vi "SweepGen.vi"(0 "#pts2":u32=21, 2 "#pts1":u32=21, 3 "Stop2":dbl=10.0 format="%.3p", 4 "Start2":dbl format="%.3p", 5 "Stop1":dbl=10.0 format="%.3p", 6 "Start1":dbl format="%.3p") -> (1 "Sweep":cluster{dbl[], dbl[]}(graph))   [LabVIEW 2022 SP3]
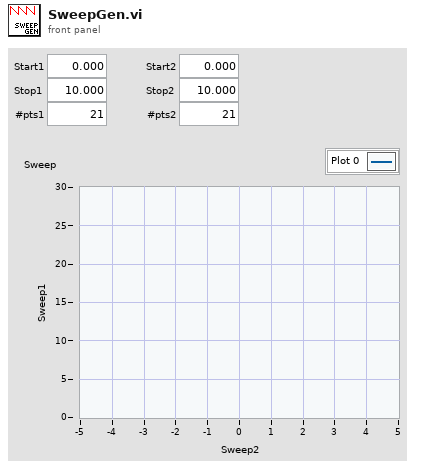
[diagram p1: front panel]
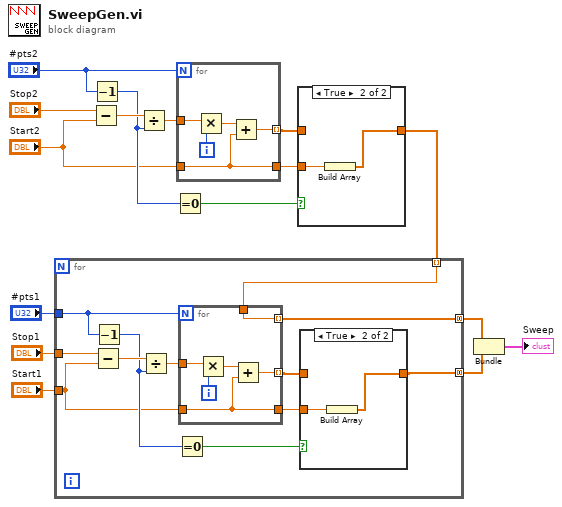
[diagram p0: block diagram]
diagram:
  n1 = Subtract(x="Stop2", y="Start2") -> (x-y=w16:dbl)
  n2 = Decrement(x="#pts2") -> (x-1=w14:u32)
  n3 = Divide(x=w16, y=w14) -> (x/y=w15:dbl)
  n4 = Equal To 0?(x=w14) -> (x = 0?=w10:bool)
  n5 = for {
    N: "#pts2" -> [_]
    tunnel: w15 -> [w21]
    tunnel: "Start2" -> [w17]
    tunnel: [w18] -> w9 mode=indexing
    tunnel: [w17] -> w8
    i -> [w20]
    n6 = Multiply(x=w21, y=w20) -> (x*y=w19:dbl)
    n7 = Add(x=w19, y=w17) -> (x+y=w18:dbl)
  }
  n8 = case shown="True" w10 {
    tunnel: [w22 w23] -> w4
    tunnel: w9 -> [w22 _]
    tunnel: w8 -> [_ w24]
    frame False {
    }
    frame True {
      n9 = Build Array(w24) -> (w23:dbl[])
    }
  }
  n10 = for {
    tunnel: "#pts1" -> [w33]
    tunnel: "Stop1" -> [w32]
    tunnel: "Start1" -> [w31]
    tunnel: w4 -> [w26] mode=indexing
    tunnel: [w27] -> w2 mode=concatenating
    tunnel: [w25] -> w3 mode=concatenating
    n11 = Subtract(x=w32, y=w31) -> (x-y=w36:dbl)
    n12 = Decrement(x=w33) -> (x-1=w34:u32)
    n13 = Divide(x=w36, y=w34) -> (x/y=w35:dbl)
    n14 = Equal To 0?(x=w34) -> (x = 0?=w30:bool)
    n15 = for {
      N: w33 -> [_]
      tunnel: w35 -> [w45]
      tunnel: w31 -> [w41]
      tunnel: [w42] -> w29 mode=indexing
      tunnel: [w41] -> w28
      tunnel: w26 -> [w40]
      tunnel: [w40] -> w25 mode=indexing
      i -> [w44]
      n16 = Multiply(x=w45, y=w44) -> (x*y=w43:dbl)
      n17 = Add(x=w43, y=w41) -> (x+y=w42:dbl)
    }
    n18 = case shown="True" w30 {
      tunnel: [w37 w38] -> w27
      tunnel: w29 -> [w37 _]
      tunnel: w28 -> [_ w39]
      frame False {
      }
      frame True {
        n19 = Build Array(w39) -> (w38:dbl[])
      }
    }
  }
  n20 = Bundle(w3, w2) -> (→"Sweep":cluster{dbl[], dbl[]})  [unwired: 1 in]
